vi "TCPReceiver Get Next Byte Length.vi"(8 "error in (no error)":errorcluster, 11 "TCPReceiver in":refnum<class "TCPReceiver.lvclass">) -> (0 "error out":errorcluster, 2 "Length":i32, 3 "TCPReceiver out":refnum<class "TCPReceiver.lvclass">)   [LabVIEW 2019, in "TCPReceiver.lvclass"]
uses:
  TCPReceiver.lvclass
  TCPReceiver.lvclass/TCPReceiver.ctl
  TCPPacket/TCPPacket.lvclass
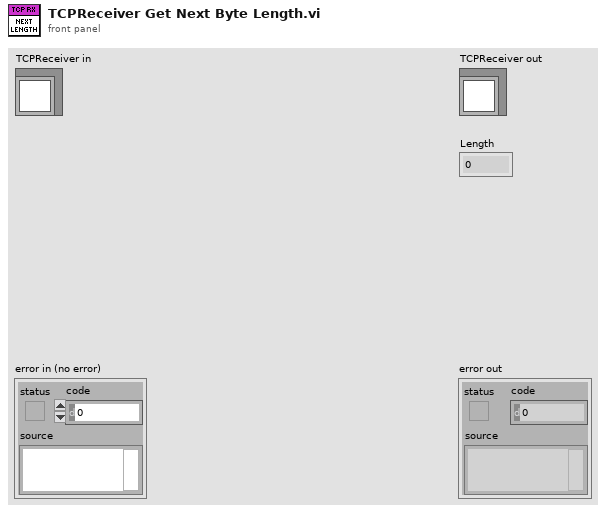
[diagram p1: front panel]
types:
  T1 = typedef "TCPReceiver.lvclass/TCPReceiver Progress STYP.ctl" = cluster{"HeaderSize?":bool, "Header?":bool, "Body?":bool}
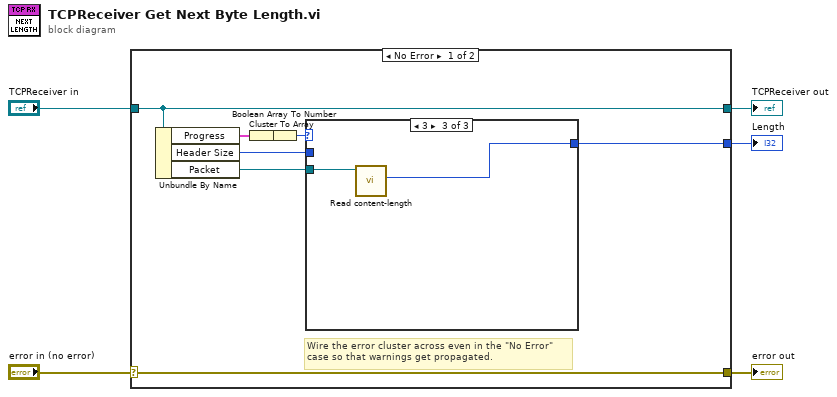
[diagram p0: block diagram]
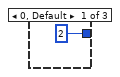
[diagram p2: hidden frame]
diagram:
  n1 = case shown="No Error" "error in (no error)" {
    selector: "error in (no error)" -> [w13 w19]
    tunnel: [w13 w19] -> w4
    tunnel: [w12 w18] -> w2
    tunnel: "TCPReceiver in" -> [w12 w18]
    tunnel: [w8 _] -> w1
    frame No Error {
      # "Wire the error cluster across even in the \"No Error\"\ncase so that warnings get propagated."
      n2 = Unbundle By Name(w12) -> ("Progress"=w11:T1, "Header Size"=w7:u16, "Packet"=w6:refnum<class "TCPPacket.lvclass">)
      n3 = Cluster To Array(cluster=w11) -> (array=w10:bool[])
      n4 = Boolean Array To Number(Boolean array=w10) -> (number=w9:u32)
      n5 = case shown="3" w9 {
        tunnel: [2 w15 w16] -> w8
        tunnel: w7 -> [_ w15 _]
        tunnel: w6 -> [_ _ w17]
        frame 0, Default {
        }
        frame 1 {
        }
        frame 3 {
          n6 = call-dynamic "Read content-length.vi"("TCPPacket in"=w17) -> ("content-length"=w16:u32)  [unwired: 8 in, 2 out]
        }
      }
    }
    frame Error {
    }
  }
  "error out" <- w4
  "TCPReceiver out" <- w2
  "Length" <- w1
